vi "Create BooleanMsg.vi"(8 "error in (no error)":errorcluster, 10 "Message Data":bool, 11 "Message Name":string) -> (0 "error out":errorcluster, 3 "BooleanMsg out":refnum<class "BooleanMsg.lvclass">)   [LabVIEW 2013, in "LapDog.Messaging.v3.NativeTypes.lvlib" / "BooleanMsg.lvclass"]
doc: "Returns a BooleanMsg object with the given name.\n\nThis method executes regardless of the error in state."
uses:
  BooleanMsg.lvclass
  LapDog.Messaging/Message/Message.lvclass
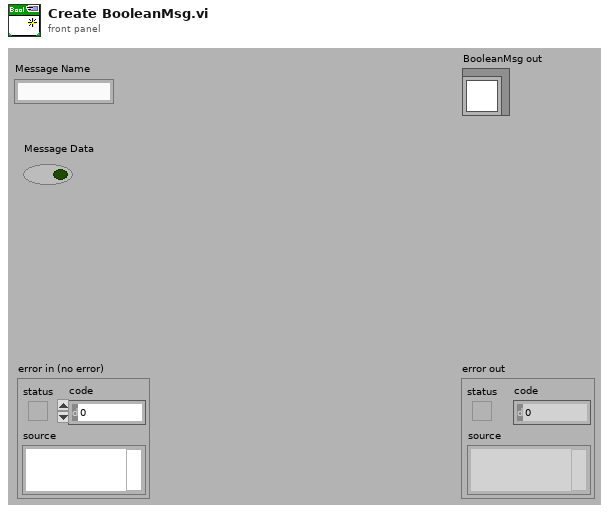
[diagram p1: front panel]
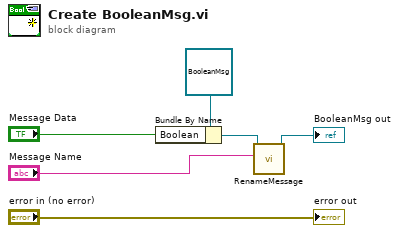
[diagram p0: block diagram]
diagram:
  n1 = Bundle By Name(cluster=refnum<class "BooleanMsg.lvclass"> refnum ("BooleanMsg in"), "Boolean"="Message Data") -> (w3:refnum<class "BooleanMsg.lvclass">)
  n2 = call "RenameMessage.vi"("Message Name"="Message Name", "Message in"=w3) -> ("Message out"=→"BooleanMsg out":refnum<class "BooleanMsg.lvclass">)  [unwired: 8 in, 1 out]
  "error out" <- "error in (no error)"
